vi "EmptyString.vi"() -> ()   [LabVIEW 2019]
panel:
  out "Empty?":bool
  in  "String":string
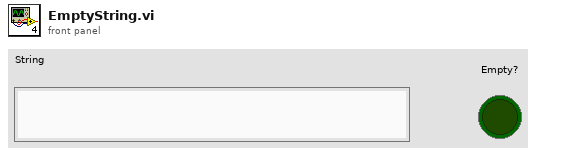
[diagram p1: front panel]
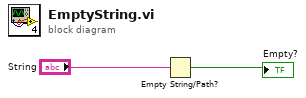
[diagram p0: block diagram]
diagram:
  n1 = Empty String/Path?(string/path="String") -> (empty?=→"Empty?":bool)
